vi "SendParameters.vi"(11 "FPGA in":refnum<queue>) -> (3 "FPGA out":refnum<queue>)   [LabVIEW 2019, in "FPGA.lvlib"]
uses:
  FPGA.lvlib
  FPGA.ctl
  Commands.ctl
panel:
  out "data string 4":string
  out "Configured":bool
  out "data string 3":string
  out "data string 2":string
  out "data string":string
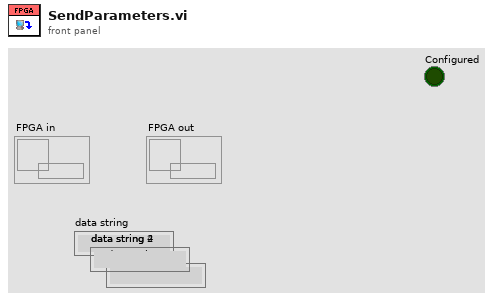
[diagram p1: front panel]
types:
  T1 = typedef "FPGA.lvlib/FPGA.ctl" = cluster{"Start freq. [Hz]":dbl, "Sweep duration [s]":dbl, "Freq. step [Hz]":dbl, "DAC Sample Rate":dbl, "ADC Sample Rate":dbl, "CMD port":u16, "DFAST port":u16, "CMD ID":refnum<k16>, "DFAST ID":refnum<k16>, "CMD error out":errorcluster, "FPGA IP":string, "DFAST error out ":errorcluster, "Stop freq. [Hz]":dbl, "Discrete sweep":bool, "Initial NCO":u32, "Difference NCO":i32, "step NCO":i64, "Final NCO":u32, "clocks for step":u32, "demodulation":bool, "NCO Phase Precision":u32, "NCO Sample Rate":dbl, "Time for step [s]":dbl, "NCO freq. resolution":dbl, "Sweep speed [Hz/s]":dbl, "Connected":bool, "Slew Rate [V/us]":dbl, "Parameters_ok":bool, "Amplitude [mVpp]":dbl, "Scale Factor":fxp<+,16,0>, "Acquiring":bool, "DAC-ADC Latency":u16, "Digital Gain":i32, "Number of steps":i32, "Averaging preferred":bool, "Filter Order":u32, "Settling":enum16{"99%", "99,9%"}}
  T2 = typedef "FPGA.lvlib/Commands.ctl" = string
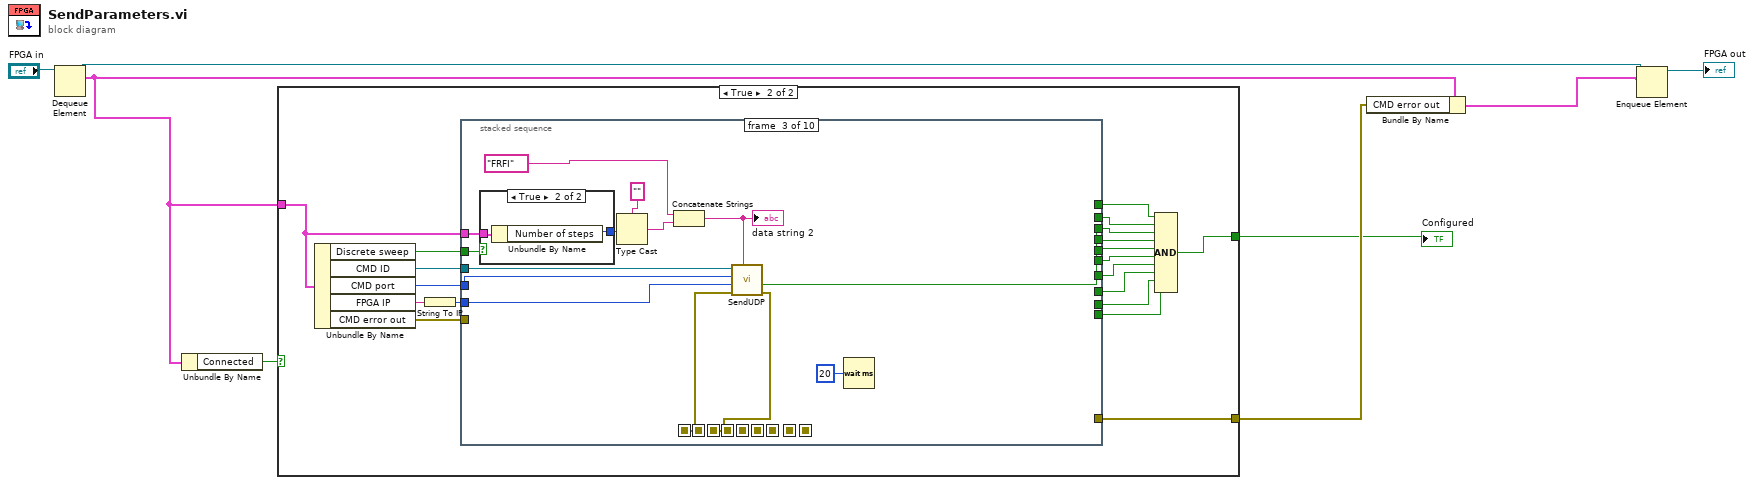
[diagram p0: block diagram]
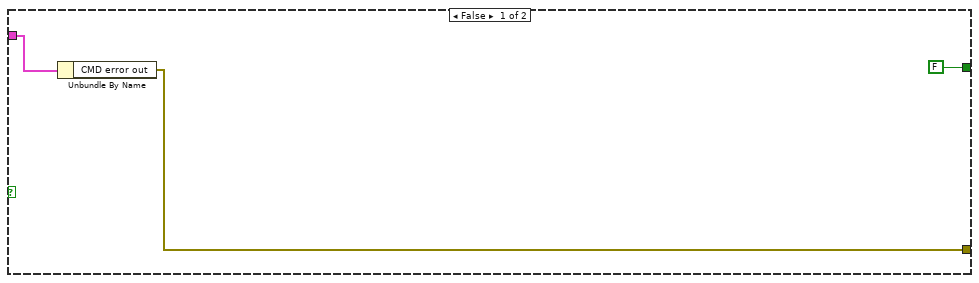
[diagram p2: hidden frame]
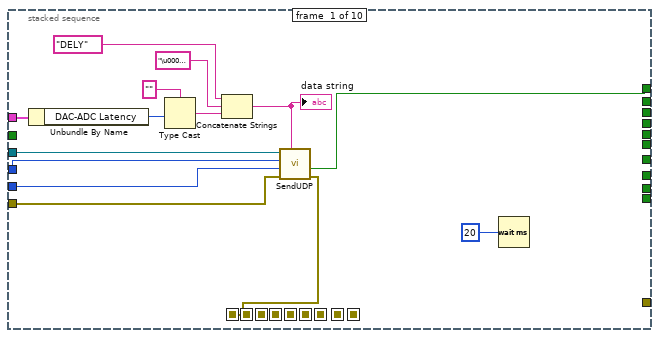
[diagram p3: hidden frame]
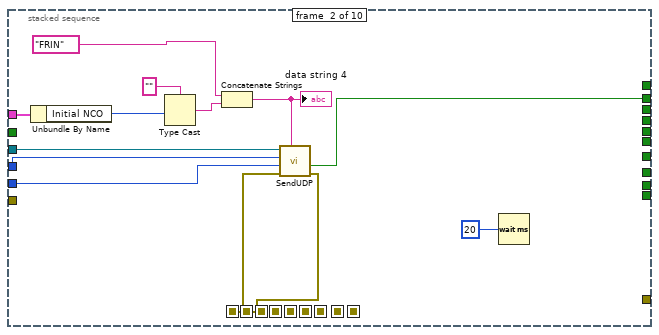
[diagram p4: hidden frame]
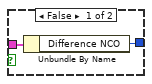
[diagram p5: hidden frame]
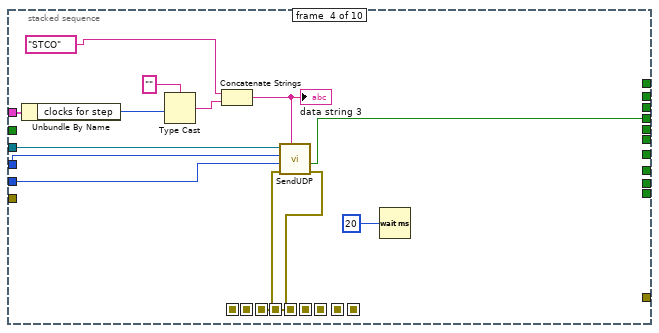
[diagram p6: hidden frame]
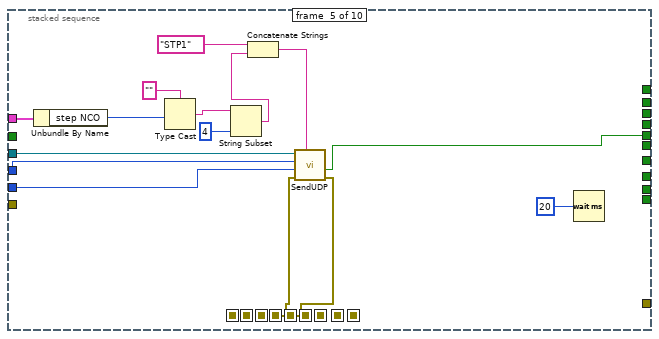
[diagram p7: hidden frame]
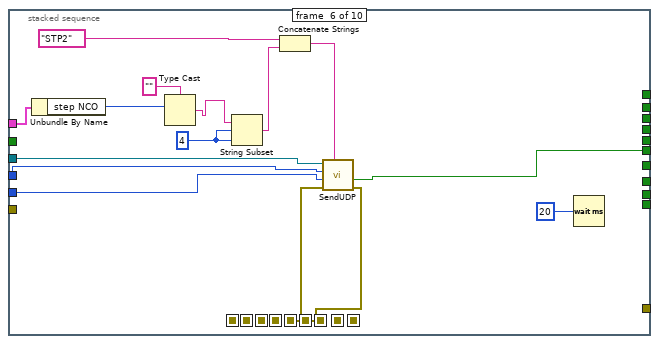
[diagram p8: hidden frame]
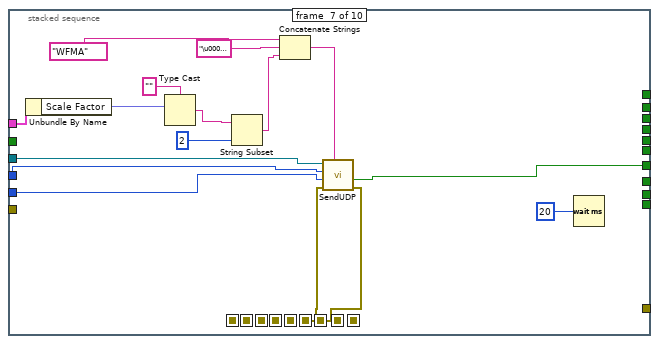
[diagram p9: hidden frame]
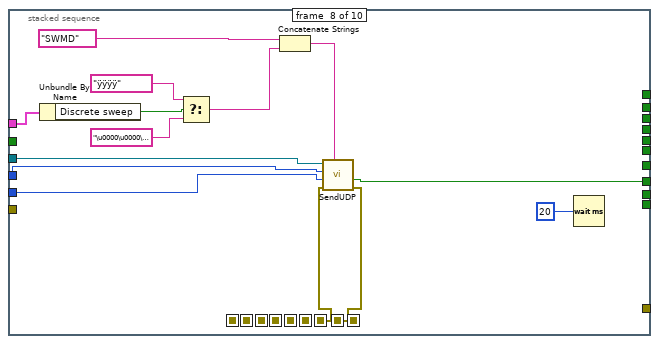
[diagram p10: hidden frame]
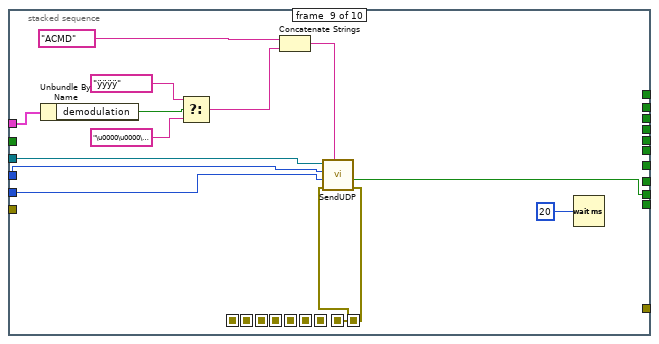
[diagram p11: hidden frame]
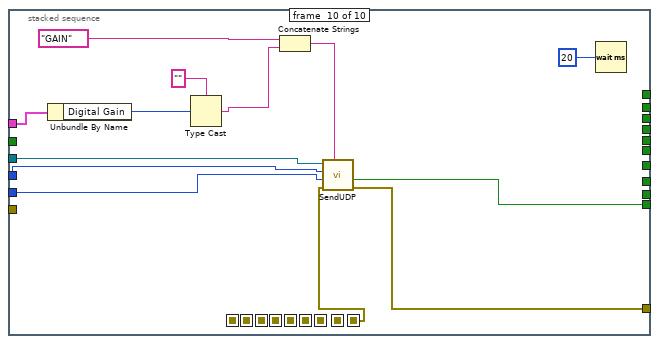
[diagram p12: hidden frame]
diagram:
  n1 = Dequeue Element(queue="FPGA in") -> (queue out=w7:refnum<queue>, element=w4:T1)  [unwired: 2 in, 2 out]
  n2 = Unbundle By Name(w4) -> ("Connected"=w5:bool)
  n3 = case shown="True" w5 {
    tunnel: w4 -> [w10 w25]
    tunnel: [w9 w24] -> w2
    tunnel: [FALSE w19] -> w1
    frame False {
      n4 = Unbundle By Name(w10) -> ("CMD error out"=w9:errorcluster)
    }
    frame True {
      n5 = Unbundle By Name(w25) -> ("Discrete sweep"=w12:bool, "CMD ID"=w29:refnum<k16>, "CMD port"=w28:u16, "FPGA IP"=w30:string, "CMD error out"=w26:errorcluster)
      n6 = String To IP(1:w30) -> (0:w27:u32)
      n7 = stacked-sequence {
        seq-local: [w36 _ _ _ _ _ _ _ _ _] -> [_ w46 w63 _ _ _ _ _ _ _]
        seq-local: [_ _ w62 _ _ _ _ _ _ _] -> [_ _ _ w79 _ _ _ _ _ _]
        seq-local: [_ _ _ w78 _ _ _ _ _ _] -> [_ _ _ _ w96 _ _ _ _ _]
        seq-local: [_ _ _ _ w89 _ _ _ _ _] -> [_ _ _ _ _ w110 _ _ _ _]
        seq-local: [_ _ _ _ _ w104 _ _ _ _] -> [_ _ _ _ _ _ w124 _ _ _]
        seq-local: [_ _ _ _ _ _ w123 _ _ _] -> [_ _ _ _ _ _ _ w136 _ _]
        seq-local: [_ _ _ _ _ _ _ w135 _ _] -> [_ _ _ _ _ _ _ _ w151 _]
        seq-local: [_ w45 _ _ _ _ _ _ _ _] -> [_ _ _ _ _ _ _ _ _ _]
        seq-local: [_ _ _ _ _ _ _ _ w149 _] -> [_ _ _ _ _ _ _ _ _ w167]
        tunnel: w29 -> [w44 w57 w71 w88 w103 w107 w126 w142 w156 w168]
        tunnel: w28 -> [w43 w56 w70 w87 w102 w108 w127 w143 w157 w169]
        tunnel: w27 -> [w42 w55 w69 w86 w101 w109 w128 w144 w158 w170]
        tunnel: w26 -> [w41 _ _ _ _ _ _ _ _ _]
        tunnel: w25 -> [w40 w54 w68 w85 w100 w118 w134 w148 w162 w175]
        tunnel: [_ w47 _ _ _ _ _ _ _ _] -> w23
        tunnel: [_ _ w64 _ _ _ _ _ _ _] -> w22
        tunnel: [_ _ _ w80 _ _ _ _ _ _] -> w21
        tunnel: [_ _ _ _ w90 _ _ _ _ _] -> w20
        tunnel: [_ _ _ _ _ _ _ _ _ w172] -> w24
        tunnel: [_ _ _ _ _ w106 _ _ _ _] -> w18
        tunnel: [_ _ _ _ _ _ _ w141 _ _] -> w16
        tunnel: [_ _ _ _ _ _ w122 _ _ _] -> w17
        tunnel: [_ _ _ _ _ _ _ _ w150 _] -> w15
        tunnel: [w31 _ _ _ _ _ _ _ _ _] -> w14
        tunnel: [_ _ _ _ _ _ _ _ _ w166] -> w13
        tunnel: w12 -> [_ _ w58 _ _ _ _ _ _ _]
        frame #0 {
          n8 = Unbundle By Name(w40) -> ("DAC-ADC Latency"=w38:u16)
          n9 = Type Cast(type="", x=w38) -> (*(type *) &x=w33:string)
          n10 = Concatenate Strings(T2 "DELY" ("Combo Box"), "\u0000\u0000" ("string"), w33) -> (w37:string)
          "data string" <- w37
          n11 = call "SendUDP.vi"("data in"=w37, "error in (no error)"=w41, "address"=w42, "port or service name"=w43, "connection ID"=w44) -> ("error out"=w36:errorcluster, "ACK"=w31:bool)  [unwired: 1 in, 4 out]
          n12 = Wait (ms)(milliseconds to wait=u32 20) -> ()  [unwired: 1 out]
        }
        frame #1 {
          n13 = Unbundle By Name(w54) -> ("Initial NCO"=w51:u32)
          n14 = Type Cast(type="", x=w51) -> (*(type *) &x=w53:string)
          n15 = Concatenate Strings(T2 "FRIN" ("Combo Box"), w53) -> (w50:string)
          "data string 4" <- w50
          n16 = call "SendUDP.vi"("data in"=w50, "error in (no error)"=w46, "address"=w55, "port or service name"=w56, "connection ID"=w57) -> ("error out"=w45:errorcluster, "ACK"=w47:bool)  [unwired: 1 in, 4 out]
          n17 = Wait (ms)(milliseconds to wait=u32 20) -> ()  [unwired: 1 out]
        }
        frame #2 {
          n18 = case shown="True" w58 {
            tunnel: w68 -> [w73 w75]
            tunnel: [w72 w74] -> w66
            frame False {
              n19 = Unbundle By Name(w73) -> ("Difference NCO"=w72:i32)
            }
            frame True {
              n20 = Unbundle By Name(w75) -> ("Number of steps"=w74:i32)
            }
          }
          n21 = Type Cast(type="", x=w66) -> (*(type *) &x=w67:string)
          n22 = Concatenate Strings(T2 "FRFI" ("Combo Box"), w67) -> (w65:string)
          "data string 2" <- w65
          n23 = call "SendUDP.vi"("data in"=w65, "error in (no error)"=w63, "address"=w69, "port or service name"=w70, "connection ID"=w71) -> ("error out"=w62:errorcluster, "ACK"=w64:bool)  [unwired: 1 in, 4 out]
          n24 = Wait (ms)(milliseconds to wait=u32 20) -> ()  [unwired: 1 out]
        }
        frame #3 {
          n25 = Unbundle By Name(w85) -> ("clocks for step"=w82:u32)
          n26 = Type Cast(type="", x=w82) -> (*(type *) &x=w84:string)
          n27 = Concatenate Strings(T2 "STCO" ("Combo Box"), w84) -> (w81:string)
          "data string 3" <- w81
          n28 = call "SendUDP.vi"("data in"=w81, "error in (no error)"=w79, "address"=w86, "port or service name"=w87, "connection ID"=w88) -> ("error out"=w78:errorcluster, "ACK"=w80:bool)  [unwired: 1 in, 4 out]
          n29 = Wait (ms)(milliseconds to wait=u32 20) -> ()  [unwired: 1 out]
        }
        frame #4 {
          n30 = Unbundle By Name(w100) -> ("step NCO"=w98:i64)
          n31 = Type Cast(type="", x=w98) -> (*(type *) &x=w93:string)
          n32 = String Subset(string=w93, length (rest)=4 ("length (rest)")) -> (substring=w94:string)  [unwired: 1 in]
          n33 = Concatenate Strings(T2 "STP1" ("Combo Box"), w94) -> (w97:string)
          n34 = call "SendUDP.vi"("data in"=w97, "error in (no error)"=w96, "address"=w101, "port or service name"=w102, "connection ID"=w103) -> ("error out"=w89:errorcluster, "ACK"=w90:bool)  [unwired: 1 in, 4 out]
          n35 = Wait (ms)(milliseconds to wait=u32 20) -> ()  [unwired: 1 out]
        }
        frame #5 {
          w105 = 4 ("length (rest)")
          n36 = Unbundle By Name(w118) -> ("step NCO"=w116:i64)
          n37 = Type Cast(type="", x=w116) -> (*(type *) &x=w115:string)
          n38 = String Subset(string=w115, offset (0)=w105, length (rest)=w105) -> (substring=w114:string)
          n39 = Concatenate Strings(T2 "STP2" ("Combo Box"), w114) -> (w112:string)
          n40 = call "SendUDP.vi"("data in"=w112, "error in (no error)"=w110, "address"=w109, "port or service name"=w108, "connection ID"=w107) -> ("error out"=w104:errorcluster, "ACK"=w106:bool)  [unwired: 1 in, 4 out]
          n41 = Wait (ms)(milliseconds to wait=u32 20) -> ()  [unwired: 1 out]
        }
        frame #6 {
          n42 = Unbundle By Name(w134) -> ("Scale Factor"=w132:fxp<+,16,0>)
          n43 = Type Cast(type="", x=w132) -> (*(type *) &x=w131:string)
          n44 = String Subset(string=w131, length (rest)=2 ("length (rest)")) -> (substring=w121:string)  [unwired: 1 in]
          n45 = Concatenate Strings(T2 "WFMA" ("Combo Box"), "\u0000\u0000" ("string"), w121) -> (w130:string)
          n46 = call "SendUDP.vi"("data in"=w130, "error in (no error)"=w124, "address"=w128, "port or service name"=w127, "connection ID"=w126) -> ("error out"=w123:errorcluster, "ACK"=w122:bool)  [unwired: 1 in, 4 out]
          n47 = Wait (ms)(milliseconds to wait=u32 20) -> ()  [unwired: 1 out]
        }
        frame #7 {
          n48 = Unbundle By Name(w148) -> ("Discrete sweep"=w139:bool)
          n49 = Select(t="ÿÿÿÿ", s=w139, f="\u0000\u0000\u0000\u0000") -> (s? t:f=w137:string)
          n50 = Concatenate Strings(T2 "SWMD" ("Combo Box"), w137) -> (w146:string)
          n51 = call "SendUDP.vi"("data in"=w146, "error in (no error)"=w136, "address"=w144, "port or service name"=w143, "connection ID"=w142) -> ("error out"=w135:errorcluster, "ACK"=w141:bool)  [unwired: 1 in, 4 out]
          n52 = Wait (ms)(milliseconds to wait=u32 20) -> ()  [unwired: 1 out]
        }
        frame #8 {
          n53 = Unbundle By Name(w162) -> ("demodulation"=w154:bool)
          n54 = Select(t="ÿÿÿÿ", s=w154, f="\u0000\u0000\u0000\u0000") -> (s? t:f=w152:string)
          n55 = Concatenate Strings(T2 "ACMD" ("Combo Box"), w152) -> (w160:string)
          n56 = call "SendUDP.vi"("data in"=w160, "error in (no error)"=w151, "address"=w158, "port or service name"=w157, "connection ID"=w156) -> ("error out"=w149:errorcluster, "ACK"=w150:bool)  [unwired: 1 in, 4 out]
          n57 = Wait (ms)(milliseconds to wait=u32 20) -> ()  [unwired: 1 out]
        }
        frame #9 {
          n58 = Unbundle By Name(w175) -> ("Digital Gain"=w165:i32)
          n59 = Type Cast(type="", x=w165) -> (*(type *) &x=w164:string)
          n60 = Concatenate Strings(T2 "GAIN" ("Combo Box"), w164) -> (w173:string)
          n61 = call "SendUDP.vi"("data in"=w173, "error in (no error)"=w167, "address"=w170, "port or service name"=w169, "connection ID"=w168) -> ("error out"=w172:errorcluster, "ACK"=w166:bool)  [unwired: 1 in, 4 out]
          n62 = Wait (ms)(milliseconds to wait=u32 20) -> ()  [unwired: 1 out]
        }
      }
      n63 = Compound Arithmetic op=AND(w14, w23, w22, w21, w20, w18, w17, w16, w15, w13) -> (w19:bool)
    }
  }
  "Configured" <- w1
  n64 = Bundle By Name(cluster=w4, "CMD error out"=w2) -> (w3:T1)
  n65 = Enqueue Element(queue=w7, element=w3) -> (queue out=→"FPGA out":refnum<queue>)  [unwired: 2 in, 2 out]
